vi "Demo Toolbar 2.vi"() -> ()   [LabVIEW 2018]
uses:
  Toolbar.xctl
  Button_Class/Button.lvclass
  Vi_Button_Class/Vi_Button.lvclass
  Button_Class/Type Defs/Button Style.ctl
  C:/Users/gavin/Documents/LabVIEW Data/LabVIEW-Bits/XControls/Toolbar/Button_Class/Button.lvclass
panel:
  in  "Toolbar":cluster{"Index":i32, "Type":T1}(xcontrol)
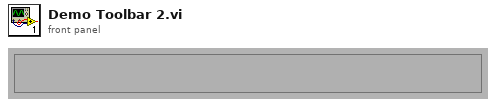
[diagram p1: front panel]
types:
  T1 = typedef "Button.lvclass/Button Events.ctl" = enum16{"Click", "Latch", "Unlatch"}
  T2 = typedef "Button.lvclass/Button Style.ctl" = enum16{"System", "Modern", "Classic", "Rounded", "Silver", "Ni Theme", "Metallic"}
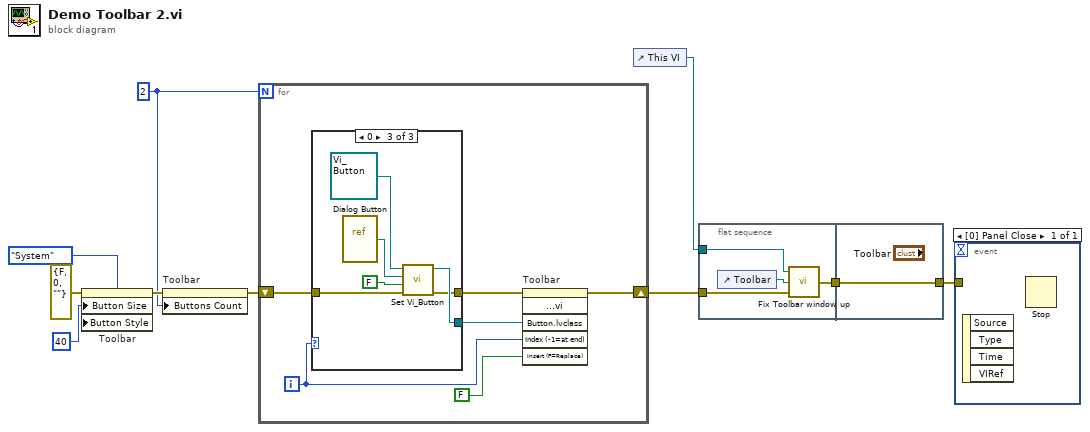
[diagram p0: block diagram]
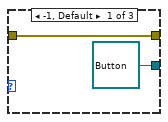
[diagram p2: hidden frame]
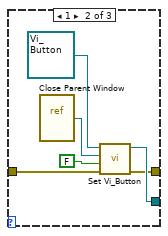
[diagram p3: hidden frame]
diagram:
  w3 = 2
  n1 = property on="Toolbar" class="Toolbar (strict)"(error in=errorcluster {"status"=FALSE, "code"=0, "source"=""} ("error out"), "Button Size"=40, "Button Style"=Button_Style."System") -> (error out=w5:errorcluster)  [unwired: 1 in, 1 out]
  n2 = property on="Toolbar" class="Toolbar (strict)"(error in=w5, "Buttons Count"=w3) -> (error out=w4:errorcluster)  [unwired: 1 in, 1 out]
  n3 = for {
    N: w3 -> [_]
    shift-right: [w11] -> w6
    shift-left: w4 -> [w15]
    i -> [w12]
    n4 = case shown="0" w12 {
      tunnel: [refnum<class "Button.lvclass"> refnum ("Button.lvclass") w23 w29] -> w16
      tunnel: w15 -> [w17 w21 w27]
      tunnel: [w17 w20 w26] -> w14
      frame -1, Default {
      }
      frame 1 {
        n5 = vi-ref "Close Parent Window.vi"() -> (w22:refnum<vi>)
        n6 = call-dynamic "Set Vi_Button.vi"("error in (no error)"=w21, "Open Window"=FALSE, "VI Refnum"=w22, "Vi_Button in"=refnum<class "Vi_Button.lvclass"> refnum ("Vi_Button.lvclass")) -> ("error out"=w20:errorcluster, "Vi_Button out"=w23:refnum<class "Vi_Button.lvclass">)  [unwired: 6 out]
      }
      frame 0 {
        n7 = vi-ref "Dialog Button.vi"() -> (w28:refnum<vi>)
        n8 = call-dynamic "Set Vi_Button.vi"("error in (no error)"=w27, "Open Window"=FALSE, "VI Refnum"=w28, "Vi_Button in"=refnum<class "Vi_Button.lvclass"> refnum ("Vi_Button.lvclass")) -> ("error out"=w26:errorcluster, "Vi_Button out"=w29:refnum<class "Vi_Button.lvclass">)  [unwired: 6 out]
      }
    }
    n9 = invoke on="Toolbar" class="Toolbar (strict)" method="Set Button From Object.vi"(error in=w14, "Button.lvclass"=w16, "Index (-1=at end)"=w12, "Insert (F=Replace)"=FALSE) -> (error out=w11:errorcluster)  [unwired: 2 in, 5 out]
  }
  n10 = control-ref of="This VI"() -> (w9:refnum<vi>)
  n11 = flat-sequence {
    tunnel: w6 -> [w34]
    tunnel: w9 -> [w33]
    tunnel: [w32] -> w7
    tunnel: [w35] -> w8
    tunnel: w7 -> [w35]
    frame #0 {
      n12 = control-ref of="Toolbar"() -> (w31:refnum<vi>)
      n13 = call "Fix Toolbar window up.vi"("Error In (no error)"=w34, "Toolbar Refnum"=w31, "Parent Vi"=w33) -> ("error out"=w32:errorcluster)
    }
    frame #1 {
    }
  }
  n14 = event shown="[0] Panel Close" {
    selector: _ -> [_]
    dyn-events: _ -> [_]
    timeout: _ -> [_]
    tunnel: w8 -> [_]
    event Panel Close {
      n15 = event-data() -> ()  [unwired: 5 out]
      n16 = Stop() -> ()  [unwired: 1 out]
    }
  }
